vi "ReceiveNorification.vi"(8 "error in (no error)":errorcluster, 11 "Balloon Notification In":refnum<class "Balloon Notification.lvclass">) -> (0 "error out":errorcluster, 3 "Balloon Notification Out":refnum<class "Balloon Notification.lvclass">)   [LabVIEW 2020, in "Balloon Notification.lvclass"]
uses:
  Balloon Notification.lvclass
  C:/Users/fflores/Documents/GitHub Projects/OOP-Concepts-in-LabVIEW/Relations Between Objects/Inheritance/Observer Pattern Example/Observer/Observer.lvclass
  <userlib>/_SmartBalloon/Balloon Generic/Aesthetics.ctl
  Observer/Observer.lvclass/Observer.ctl
  ca2ffe99-670d-442a-886b-63d2ff46782a.vi
  <userlib>/_SmartBalloon/Balloon/Text Balloon.lvclass
  C:/Program Files (x86)/National Instruments/LabVIEW 2020/user.lib/_SmartBalloon/Balloon Generic/Balloon.lvclass
  <userlib>/_SmartBalloon/Balloon/Init Balloon.vi
  <userlib>/_SmartBalloon/API/SmartBalloon Library.lvclass
  <userlib>/_SmartBalloon/Balloon Generic/Balloon.lvclass
  Observer/Observer.lvclass
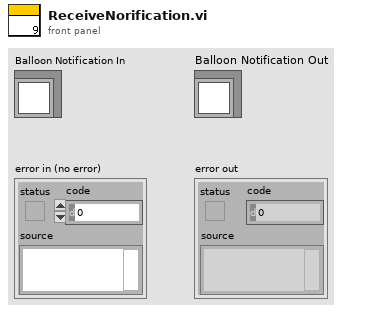
[diagram p1: front panel]
types:
  T1 = typedef "Balloon Engine.lvlib/Balloon.lvclass/Aesthetics.ctl" = cluster{"Colors":cluster{"Font Color":u32, "Panel Color":u32}, "Display Time (ms)":i32}
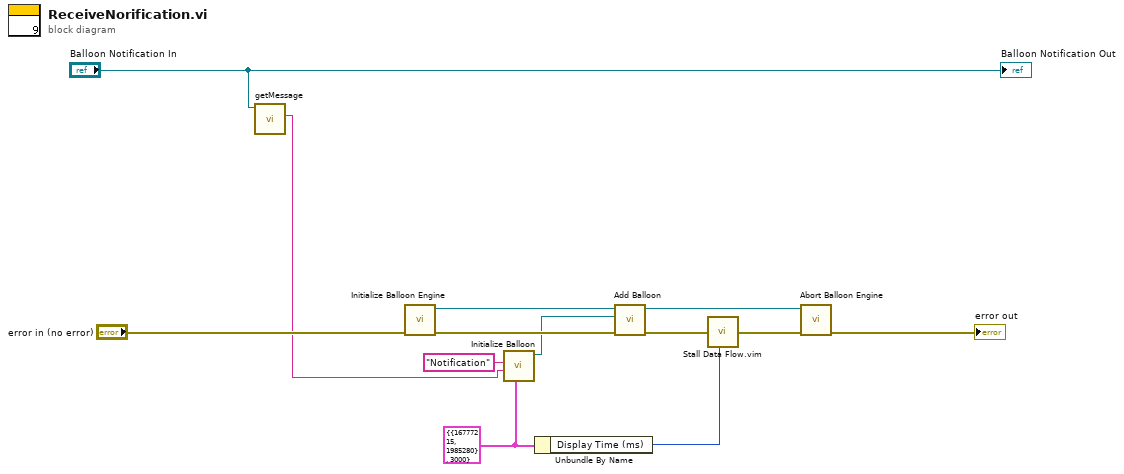
[diagram p0: block diagram]
diagram:
  w3 = T1 {"Colors"={"Font Color"=16777215, "Panel Color"=1985280}, "Display Time (ms)"=3000} ("Aesthetics")
  n1 = call "getMessage.vi"("Observer in"="Balloon Notification In") -> ("Message"=w6:string)  [unwired: 8 in, 2 out]
  n2 = call <userlib>:"Initialize Balloon Engine.vi"("error in (no error)"="error in (no error)") -> ("error out"=w10:errorcluster, "SmartBalloon Library.lvclass"=w9:refnum<class "SmartBalloon Library.lvclass">)  [unwired: 9 in]
  n3 = call-poly <userlib>:"Initialize Balloon.vi"("Aesthetics"=w3, "Body"=w6, "Title"="Notification") -> ("Balloon out"=w7:refnum<class "Text Balloon.lvclass">)  [unwired: 7 in, 1 out]
  n4 = Unbundle By Name(w3) -> ("Display Time (ms)"=w1:i32)
  n5 = call <userlib>:"Add Balloon.vi"("error in (no error)"=w10, "Next Balloon"=w7, "SmartBalloon Engine Reference"=w9) -> ("error out"=w12:errorcluster, "SmartBalloon Engine Reference out"=w4:refnum<class "SmartBalloon Library.lvclass">)  [unwired: 7 in]
  n6 = call "Stall Data Flow.vim"("value in"=w12, "milliseconds to wait"=w1) -> ("value out"=w2:errorcluster)  [unwired: 1 out]
  n7 = call <userlib>:"Abort Balloon Engine.vi"("error in (no error)"=w2, "SmartBalloon Engine Reference"=w4) -> ("error out"=→"error out":errorcluster)  [unwired: 9 in]
  "Balloon Notification Out" <- "Balloon Notification In"
